vi "send_command.vi"(4 "error in":errorcluster, 5 "Timeout ms (25000)":i32=20000, 6 "JSON Command":string, 7 "TCP Network Connection in":refnum<k5>) -> (0 "error out":errorcluster, 1 "Response":string, 2 "Success":bool, 3 "TCP Network Connection Out":refnum<k5>)   [LabVIEW 2019]
doc: "Send a command via TCP with format \"type\", \"success\", \"reference\", \"message\". This VI is used to send server commands."
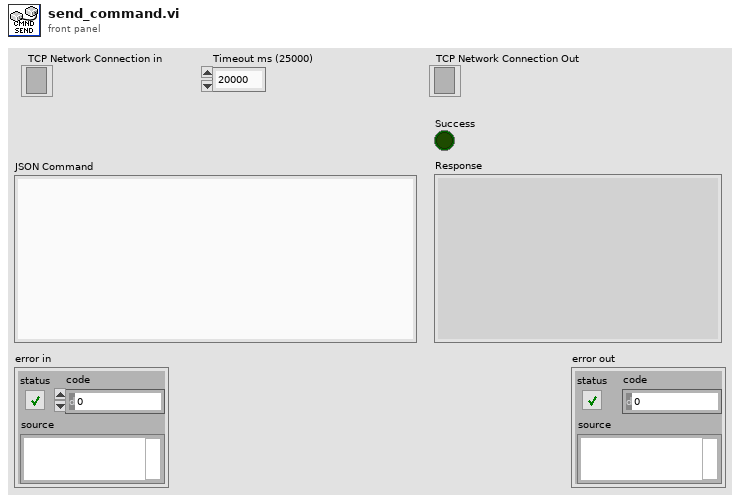
[diagram p1: front panel]
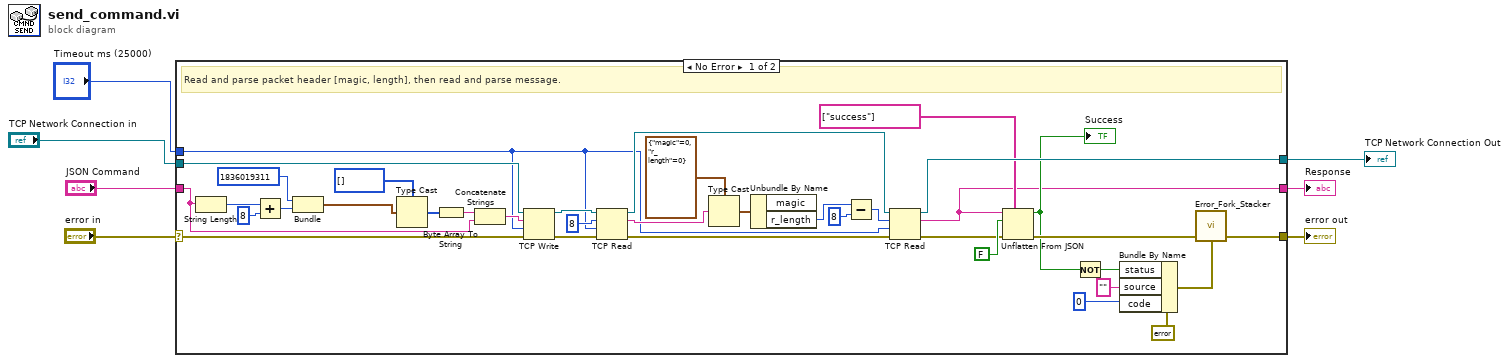
[diagram p0: block diagram]
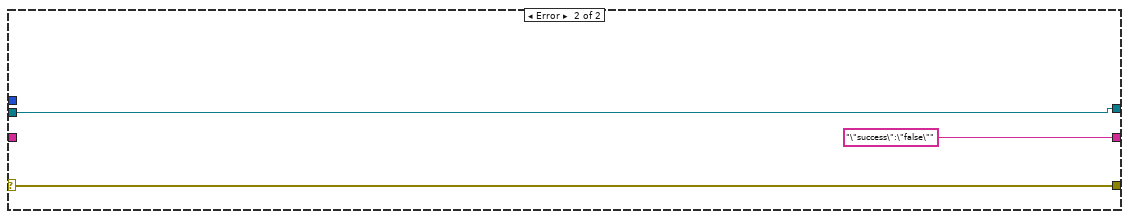
[diagram p2: hidden frame]
diagram:
  n1 = case shown="No Error" "error in" {
    selector: "error in" -> [w21 w46]
    tunnel: [w12 "\"success\":\"false\"" ("data out")] -> w7
    tunnel: "TCP Network Connection in" -> [w25 w45]
    tunnel: "JSON Command" -> [w24 _]
    tunnel: [w16 w46] -> w3
    tunnel: [w22 w45] -> w2
    tunnel: "Timeout ms (25000)" -> [w20 _]
    frame No Error {
      # "Read and parse packet header [magic, length], then read and parse message."
      n2 = String Length(string=w24) -> (length=w26:i32)
      n3 = Add(x=w26, y=u32 8) -> (x+y=w37:u32)
      n4 = Bundle(u32 1836019311, w37) -> (w42:cluster{u32, u32})  [unwired: 1 in]
      n5 = Type Cast(type=u8[] [], x=w42) -> (*(type *) &x=w40:u8[])
      n6 = Byte Array To String(unsigned byte array=w40) -> (string=w36:string)
      n7 = Concatenate Strings(w36, w24) -> (w23:string)
      n8 = TCP Write(connection ID=w25, data in=w23, error in (no error)=w21, 9:w20) -> (connection ID out=w43:refnum<k5>, error out=w44:errorcluster)  [unwired: 1 out]
      n9 = TCP Read(connection ID=w43, bytes to read=8, error in (no error)=w44, 9:w20) -> (connection ID out=w30:refnum<k5>, data out=w35:string, error out=w31:errorcluster)  [unwired: 1 in]
      n10 = Type Cast(type=cluster{"magic":u32, "r_length":u32} {"magic"=0, "r_length"=0}, x=w35) -> (*(type *) &x=w34:cluster{"magic":u32, "r_length":u32})
      n11 = Unbundle By Name(w34) -> ("r_length"=w32:u32)  [unwired: 1 out]
      n12 = Subtract(x=w32, y=u32 8) -> (x-y=w33:u32)
      n13 = TCP Read(connection ID=w30, bytes to read=w33, error in (no error)=w31, 9:w20) -> (connection ID out=w22:refnum<k5>, data out=w12:string, error out=w15:errorcluster)  [unwired: 1 in]
      n14 = Unflatten From JSON(path=string[] ["success"], JSON string=w12, type and defaults=FALSE ("strict validation? (F)"), error in (no error)=w15) -> (value=w14:bool, error out=w17:errorcluster)  [unwired: 3 in]
      "Success" <- w14
      n15 = Not(x=w14) -> (.not. x?=w13:bool)
      n16 = Bundle By Name(cluster=errorcluster {"status"=FALSE, "code"=0, "source"=""} ("error out"), "status"=w13, "source"="", "code"=0) -> (w10:errorcluster)
      n17 = call "Error_Fork_Stacker.vi"("Error Fork B"=w10, "Error Fork A"=w17) -> ("Error Out"=w16:errorcluster)  [unwired: 2 in]
    }
    frame Error {
    }
  }
  "error out" <- w3
  "Response" <- w7
  "TCP Network Connection Out" <- w2
